vi "Class Constants.vi"   [LabVIEW 2019]
doc: "This VI insures our classes are all complied in the application."
uses:
  Classes/Cargo/Cargo Concrete/Cargo Concrete.lvclass
  Classes/Cargo/Cargo PacBot/Cargo PacBot.lvclass
  Classes/Cargo/Cargo Simulated/Cargo Simulated.lvclass
  Classes/Cargo/Cargo.lvclass
  Classes/DriveOld/Drive.lvclass
  Classes/DriveOld/Pod Drive/Pod Drive.lvclass
  Classes/DriveOld/Simulated Drive/Simulated Drive.lvclass
  Classes/Drive/Tank Drive/CTRE Drive/CTRE Drive.lvclass
  Classes/Drive/Tank Drive/CTRE Drive/Falcon500/Falcon500.lvclass
  Classes/Drive/Tank Drive/CTRE Drive/TalonSRX/TalonSRX.lvclass
  Classes/Drive/Tank Drive/Tank Drive.lvclass
  Classes/Elevator/Elevator Arm/Elevator Arm.lvclass
  Classes/Elevator/Elevator Simulated/Elevator Simulated.lvclass
  Classes/Elevator/Elevator.lvclass
  Classes/Elevator/Elevator Linear/Elevator Linear.lvclass
  Classes/Hatch/Hatch Concrete/Hatch Concrete.lvclass
  Classes/Hatch/Hatch Simulated/Hatch Simulated.lvclass
  Classes/Hatch/Hatch.lvclass
  Classes/Pnematics control/Pneumatics.lvclass
  Classes/Pnematics control/Solenoids/Solenoids.lvclass
  Classes/Pnematics control/Solenoids/SingleSolenoid.lvclass
  Classes/Pnematics control/Solenoids/DoubleSolenoid.lvclass
  Classes/Vision/Vision.lvclass
  Classes/Joysticks/Two Drivers/Two Drivers.lvclass
  Classes/Joysticks/One Driver/One Driver.lvclass
  Classes/Joysticks/Joysticks.lvclass
  Classes/Configuration File/Configuration File.lvclass
  Classes/Robot/Outlaw/Outlaw.lvclass
  Classes/Robot/Robot.lvclass
  Classes/Robot/Panzer/Panzer.lvclass
  Classes/Control Panel/Control Panel.lvclass
  Classes/Climber/Climber.lvclass
  Classes/Climber/Scissor/ScissorClimber.lvclass
  Classes/Turret/Turret.lvclass
  Classes/PowerCellHandler/Power Cell Handler.lvclass
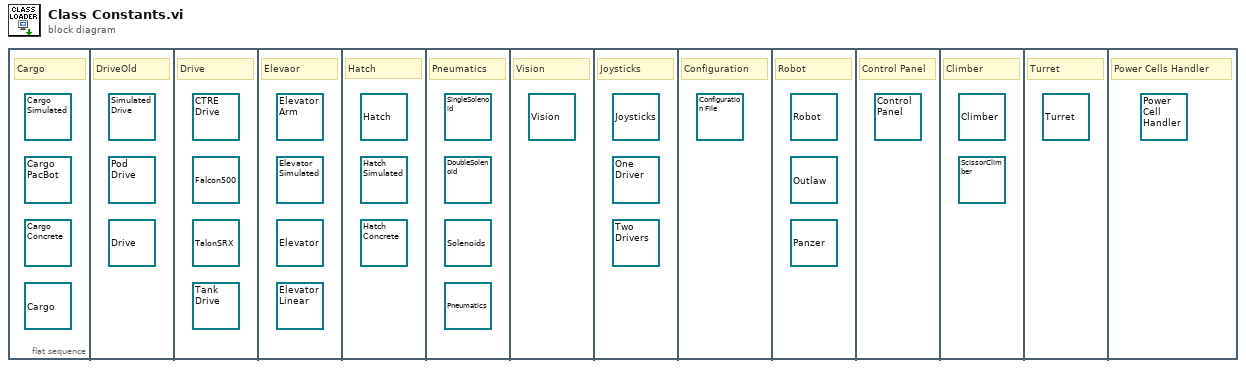
[diagram p0: block diagram]
diagram:
  n1 = flat-sequence {
    frame #0 {
      (unwired) refnum<class "Cargo.lvclass"> refnum ("Cargo.lvlib:Cargo.lvclass")
      (unwired) refnum<class "Cargo Simulated.lvclass"> refnum ("Cargo.lvlib:Cargo Simulated.lvclass")
      (unwired) refnum<class "Cargo PacBot.lvclass"> refnum ("Cargo.lvlib:Cargo PacBot.lvclass")
      (unwired) refnum<class "Cargo Concrete.lvclass"> refnum ("Cargo.lvlib:Cargo Concrete.lvclass")
      # "Cargo"
    }
    frame #1 {
      (unwired) refnum<class "Simulated Drive.lvclass"> refnum ("Drive.lvlib:Simulated Drive.lvclass")
      (unwired) refnum<class "Pod Drive.lvclass"> refnum ("Drive.lvlib:Pod Drive.lvclass")
      (unwired) refnum<class "Drive.lvclass"> refnum ("Drive.lvlib:Drive.lvclass")
      # "DriveOld"
    }
    frame #2 {
      (unwired) refnum<class "Tank Drive.lvclass"> refnum ("Drive.lvlib:Tank Drive.lvclass")
      (unwired) refnum<class "TalonSRX.lvclass"> refnum ("Drive.lvlib:TalonSRX.lvclass")
      (unwired) refnum<class "Falcon500.lvclass"> refnum ("Drive.lvlib:Falcon500.lvclass")
      (unwired) refnum<class "CTRE Drive.lvclass"> refnum ("Drive.lvlib:CTRE Drive.lvclass")
      # "Drive"
    }
    frame #3 {
      (unwired) refnum<class "Elevator Linear.lvclass"> refnum ("Elevator.lvlib:Elevator Linear.lvclass")
      (unwired) refnum<class "Elevator.lvclass"> refnum ("Elevator.lvlib:Elevator.lvclass")
      (unwired) refnum<class "Elevator Simulated.lvclass"> refnum ("Elevator.lvlib:Elevator Simulated.lvclass")
      (unwired) refnum<class "Elevator Arm.lvclass"> refnum ("Elevator.lvlib:Elevator Arm.lvclass")
      # "Elevaor"
    }
    frame #4 {
      (unwired) refnum<class "Hatch.lvclass"> refnum ("Hatch.lvlib:Hatch.lvclass")
      (unwired) refnum<class "Hatch Simulated.lvclass"> refnum ("Hatch.lvlib:Hatch Simulated.lvclass")
      (unwired) refnum<class "Hatch Concrete.lvclass"> refnum ("Hatch.lvlib:Hatch Concrete.lvclass")
      # "Hatch"
    }
    frame #5 {
      (unwired) refnum<class "DoubleSolenoid.lvclass"> refnum ("Pneumatics control.lvlib:DoubleSolenoid.lvclass")
      (unwired) refnum<class "SingleSolenoid.lvclass"> refnum ("Pneumatics control.lvlib:SingleSolenoid.lvclass")
      (unwired) refnum<class "Solenoids.lvclass"> refnum ("Pneumatics control.lvlib:Solenoids.lvclass")
      (unwired) refnum<class "Pneumatics.lvclass"> refnum ("Pneumatics control.lvlib:Pneumatics.lvclass")
      # "Pneumatics"
    }
    frame #6 {
      (unwired) refnum<class "Vision.lvclass"> refnum ("Vision.lvlib:Vision.lvclass")
      # "Vision"
    }
    frame #7 {
      (unwired) refnum<class "Joysticks.lvclass"> refnum ("Joysticks.lvlib:Joysticks.lvclass")
      (unwired) refnum<class "One Driver.lvclass"> refnum ("Joysticks.lvlib:One Driver.lvclass")
      (unwired) refnum<class "Two Drivers.lvclass"> refnum ("Joysticks.lvlib:Two Drivers.lvclass")
      # "Joysticks"
    }
    frame #8 {
      (unwired) refnum<class "Configuration File.lvclass"> refnum ("Configuration File.lvlib:Configuration File.lvclass")
      # "Configuration"
    }
    frame #9 {
      (unwired) refnum<class "Panzer.lvclass"> refnum ("Robot:Panzer.lvclass")
      (unwired) refnum<class "Robot.lvclass"> refnum ("Robot:Robot.lvclass")
      (unwired) refnum<class "Outlaw.lvclass"> refnum ("Robot:Outlaw.lvclass")
      # "Robot"
    }
    frame #10 {
      (unwired) refnum<class "Control Panel.lvclass"> refnum ("Control Panel.lvlib:Control Panel.lvclass")
      # "Control Panel"
    }
    frame #11 {
      (unwired) refnum<class "ScissorClimber.lvclass"> refnum ("Climber.lvlib:ScissorClimber.lvclass")
      (unwired) refnum<class "Climber.lvclass"> refnum ("Climber.lvlib:Climber.lvclass")
      # "Climber"
    }
    frame #12 {
      (unwired) refnum<class "Turret.lvclass"> refnum ("Turret.lvlib:Turret.lvclass")
      # "Turret"
    }
    frame #13 {
      (unwired) refnum<class "Power Cell Handler.lvclass"> refnum ("Power Cell Handler.lvlib:Power Cell Handler.lvclass")
      # "Power Cells Handler"
    }
  }
